vi "CSDB_SVEdit.main.vi"() -> ()   [LabVIEW 2014, in "CSDB_SVEdit.lvlib"]
doc: "Main VI of the Shared Variable Editor"
uses:
  CSDB_SVEdit.lvlib
panel:
  in  "dryRun":bool
  in  "showModifyProperty":bool
  in  "showSelected":bool
  in  "saveFile":bool
  in  "loadFile":bool
  in  "Undo":bool
  in  "doIt":bool
  in  "modifyValue":string
  in  "\"modifyValue\" preSelect":u16(ring)
  in  "usingAction":u16(ring)=3 items=["N/A", "append", "prefix", "replace"]
  in  "byValue":string
  in  "\"byValue\" preSelect":u16(ring)
  in  "modifyProperty":u16(ring)
  in  "\"selectValue\" preSelect":u16(ring)
  in  "selectValue":string
  in  "selectProperty":u16(ring)
  in  "sharedVariables":string[][](table)
  in  "exit":bool
  out "error out":errorcluster
  in  "error in (no error)":errorcluster
  in  "CSVPath":path
  # "if"
  # "Use \"selectProperty\" and \n\"selectName\" to select \nShared Variables (ROWS)"
  # "Use \"modifyProperty\" and \n\"modifyName\" to select values\nfor change (CELLS in a COLUMN)"
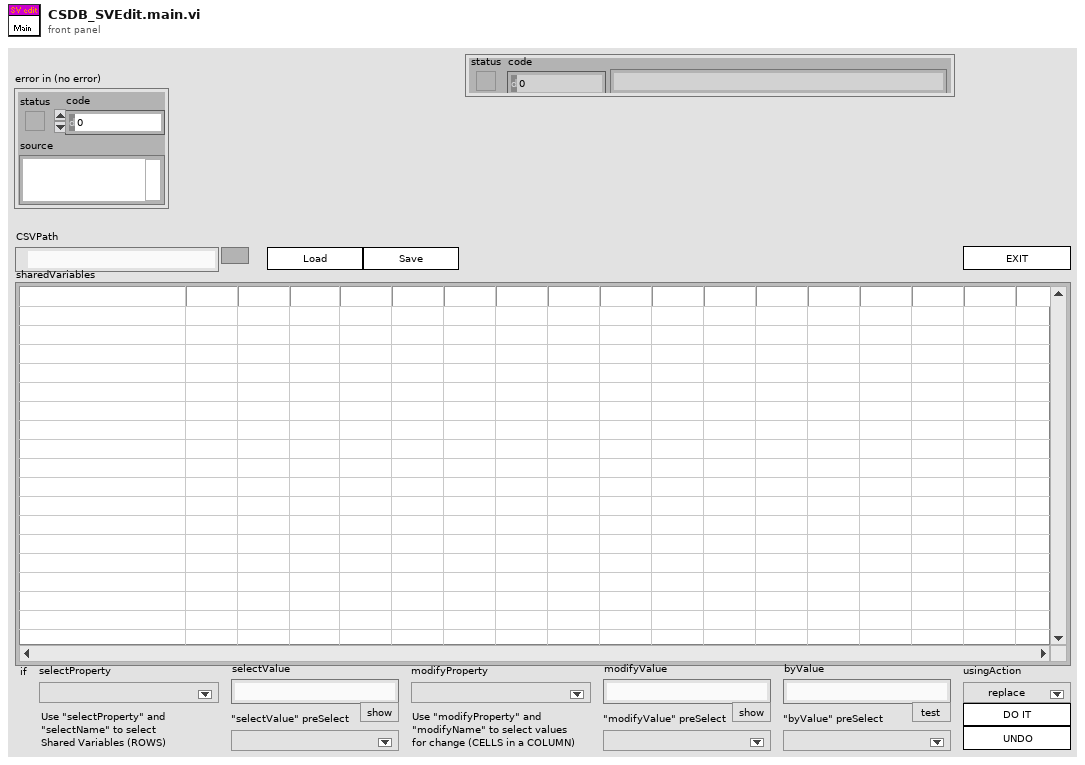
[diagram p1: front panel]
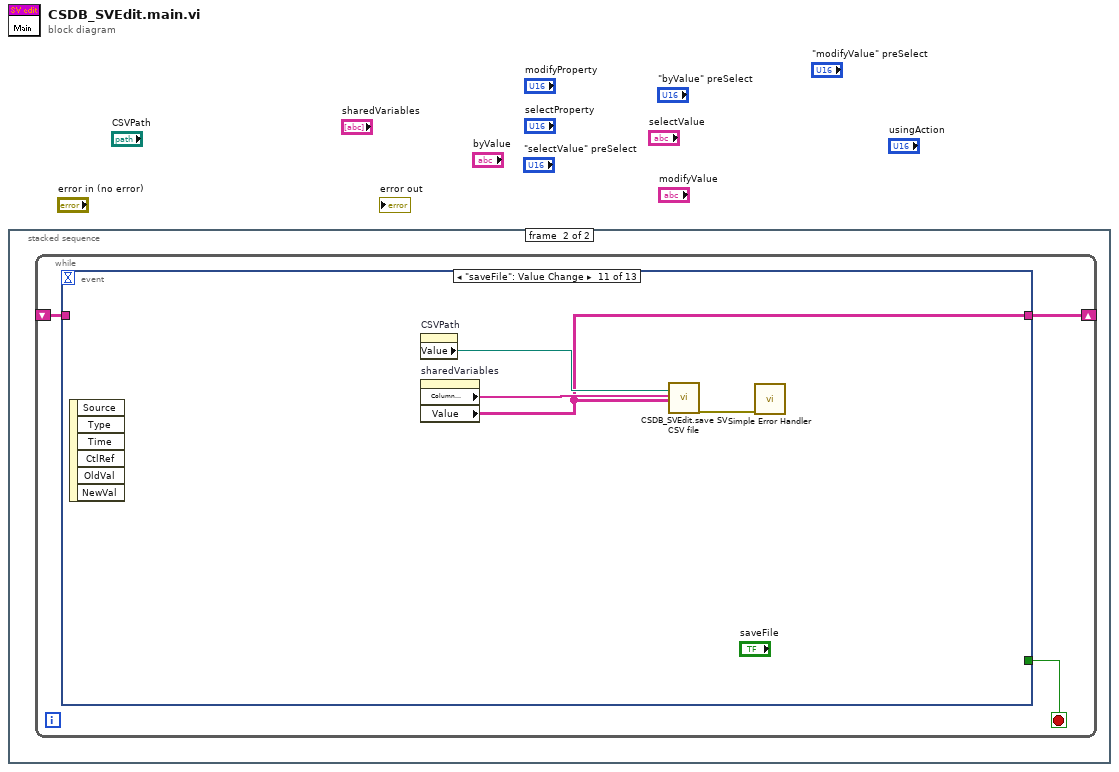
[diagram p0: block diagram]
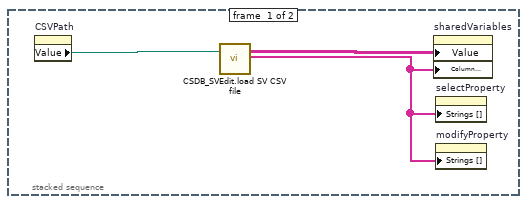
[diagram p2: hidden frame]
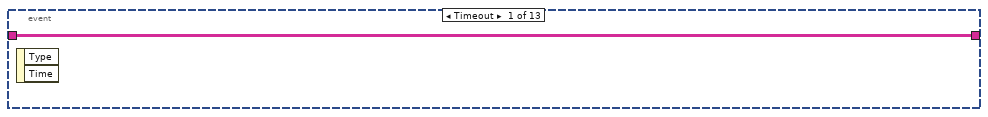
[diagram p3: hidden frame]
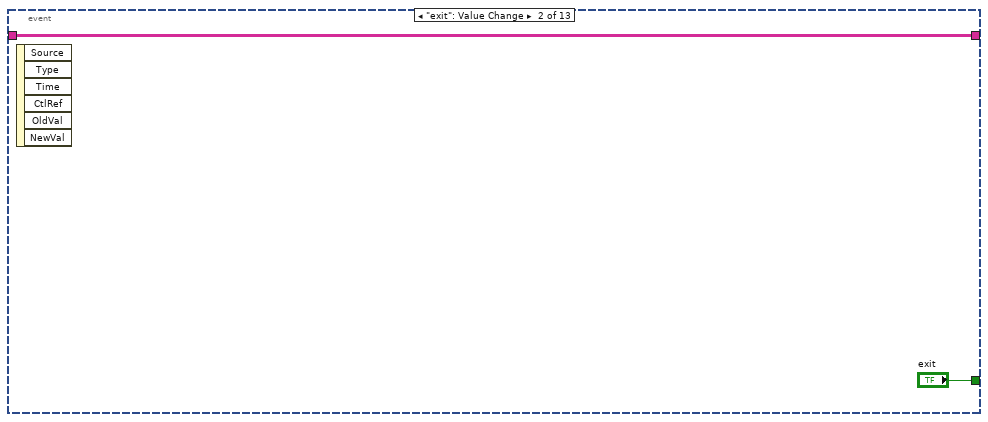
[diagram p4: hidden frame]
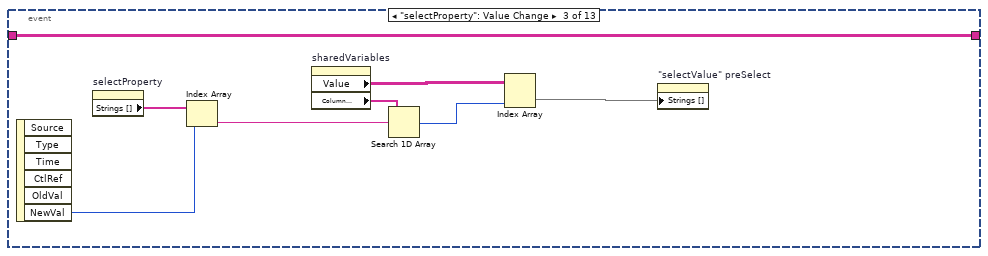
[diagram p5: hidden frame]
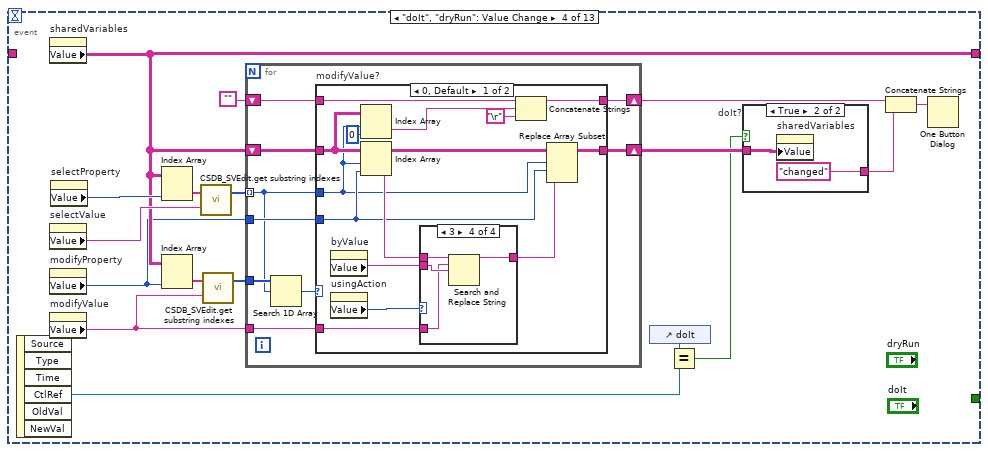
[diagram p6: hidden frame]
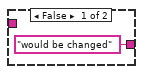
[diagram p7: hidden frame]
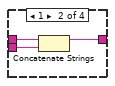
[diagram p9: hidden frame]
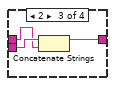
[diagram p10: hidden frame]
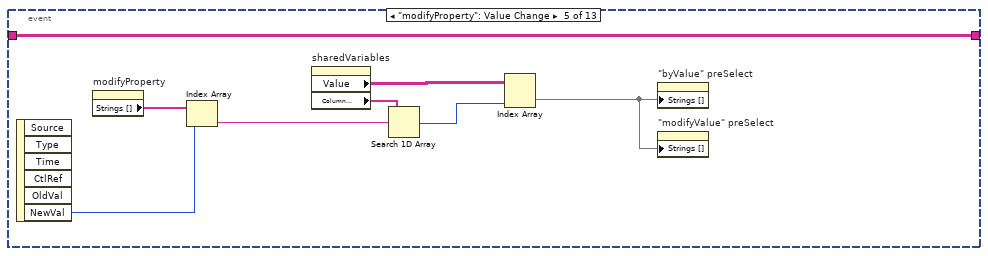
[diagram p12: hidden frame]
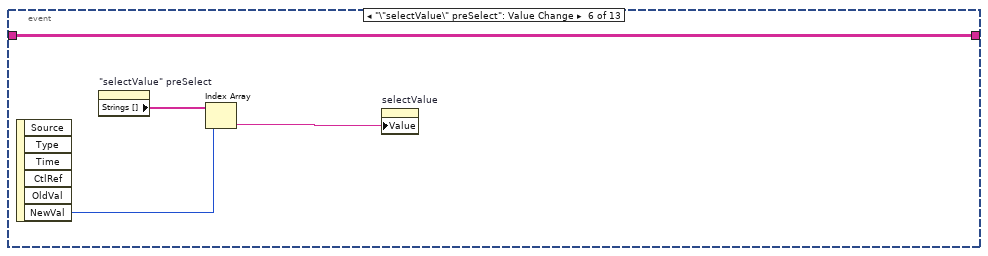
[diagram p13: hidden frame]
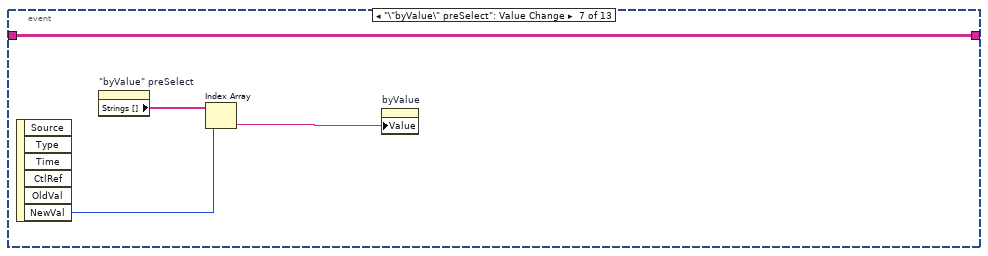
[diagram p14: hidden frame]
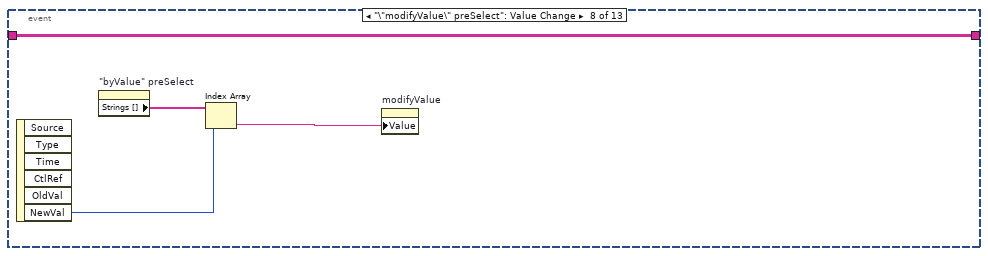
[diagram p15: hidden frame]
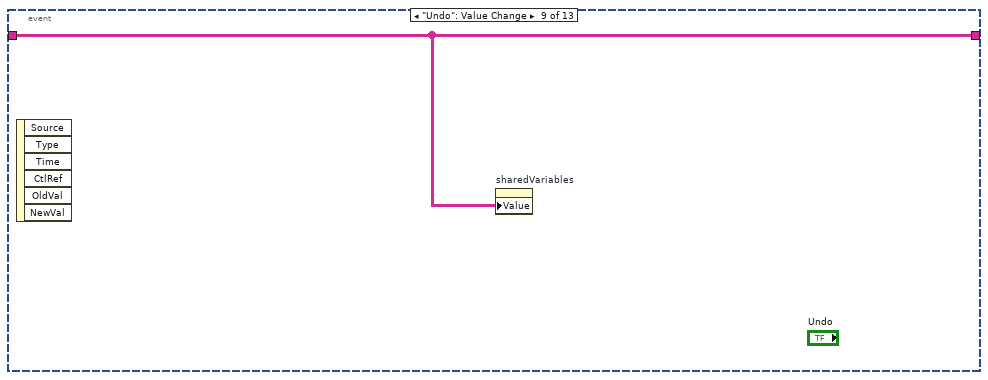
[diagram p16: hidden frame]
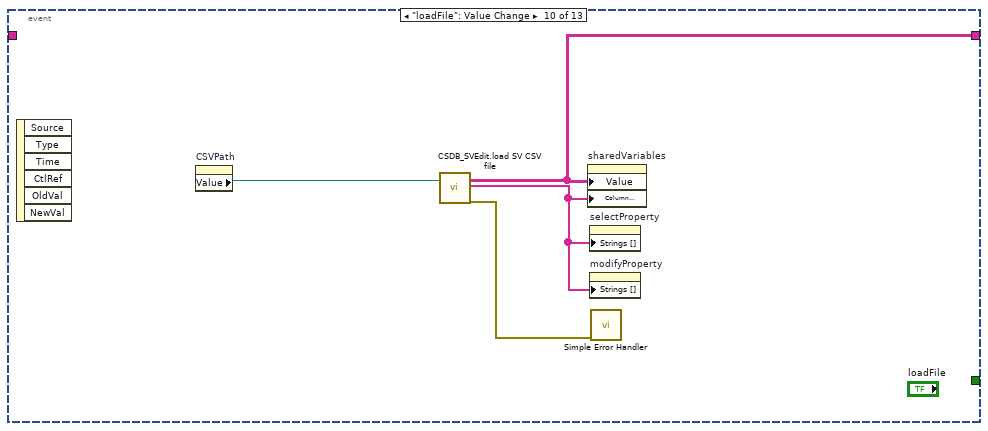
[diagram p17: hidden frame]
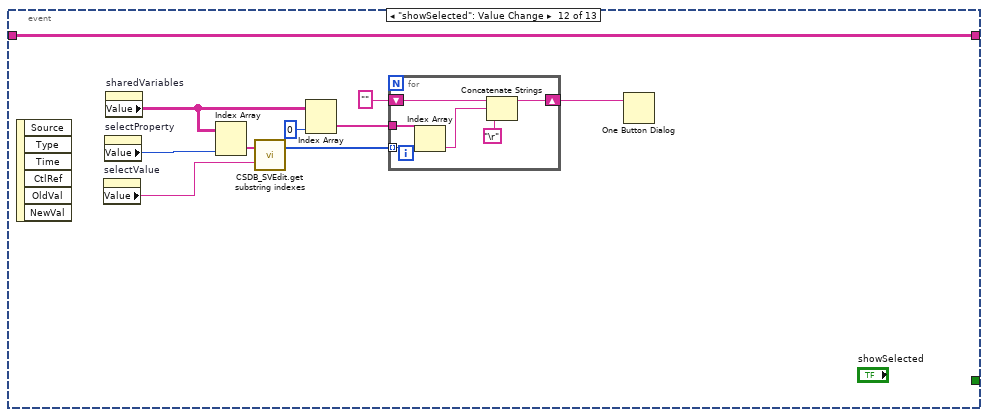
[diagram p18: hidden frame]
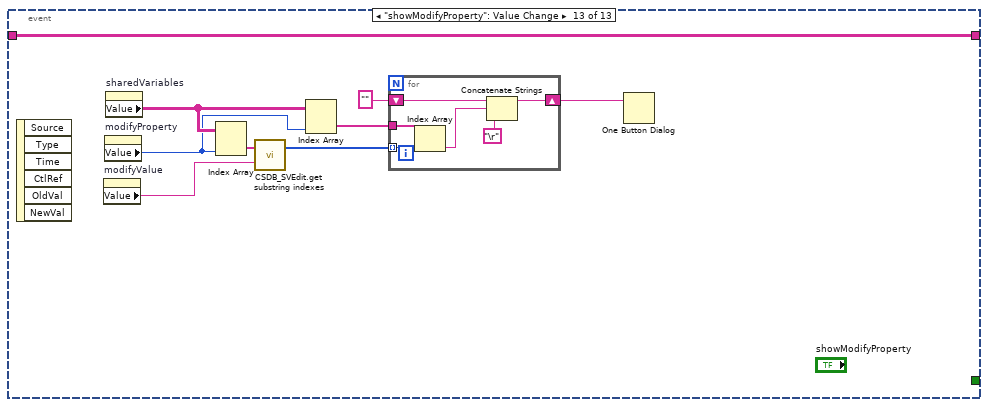
[diagram p19: hidden frame]
diagram:
  n1 = stacked-sequence {
    frame #0 {
      n2 = property on="CSVPath" class="Path"() -> ("Value"=w1:path)  [unwired: 2 in, 2 out]
      n3 = call "CSDB_SVEdit.load SV CSV file.vi"("CSVPath"=w1) -> ("SVValues"=w3:string[][], "SVHeader"=w2:string[])  [unwired: 16 in, 1 out]
      n4 = property on="sharedVariables" class="Tbl (strict)"("Value"=w3, "Column Headers[]"=w2) -> ()  [unwired: 2 in, 2 out]
      n5 = property on="selectProperty" class="Ring (strict)"("Strings []"=w2) -> ()  [unwired: 2 in, 2 out]
      n6 = property on="modifyProperty" class="Ring (strict)"("Strings []"=w2) -> ()  [unwired: 2 in, 2 out]
    }
    frame #1 {
      n7 = while {
        shift-right: [w5] -> _
        shift-left: _ -> [w4]
        stop <- w6 stop-if-true
        n8 = event shown="[10] \"saveFile\": Value Change" {
          selector: _ -> [_ _ _ _ _ _ _ _ _ _ _ _ _]
          dyn-events: _ -> [_ _ _ _ _ _ _ _ _ _ _ _ _]
          timeout: _ -> [_ _ _ _ _ _ _ _ _ _ _ _ _]
          tunnel: [_ "exit" _ _ _ _ _ _ _ _ _ _ _] -> w6
          tunnel: [w7 w8 w10 w28 w74 w82 w86 w90 w94 w96 w99 w112 w127] -> w5
          tunnel: w4 -> [w7 w8 w10 _ w74 w82 w86 w90 w94 _ _ w112 w127]
          event Timeout {
            n9 = event-data() -> ()  [unwired: 1 in, 2 out]
          }
          event "exit": Value Change {
            n10 = event-data() -> ()  [unwired: 1 in, 6 out]
          }
          event "selectProperty": Value Change {
            n11 = event-data() -> ("NewVal"=w16:u16)  [unwired: 1 in, 5 out]
            n12 = property on="selectProperty" class="Ring (strict)"() -> ("Strings []"=w17:string[])  [unwired: 2 in, 2 out]
            n13 = Index Array(array=w17, index=w16) -> (element=w15:string)
            n14 = property on="sharedVariables" class="Tbl (strict)"() -> ("Value"=w13:string[][], "Column Headers[]"=w14:string[])  [unwired: 2 in, 2 out]
            n15 = Search 1D Array(1D array=w14, element=w15) -> (index of element=w12:i32)  [unwired: 1 in]
            n16 = Index Array(array=w13, index (col)=w12) -> (element=w11:string[])  [unwired: 1 in]
            n17 = property on="\"selectValue\" preSelect" class="Ring (strict)"("Strings []"=w11) -> ()  [unwired: 2 in, 2 out]
          }
          event "doIt", "dryRun": Value Change {
            n18 = event-data() -> ("CtlRef"=w23:refnum<vi>)  [unwired: 1 in, 5 out]
            n19 = property on="sharedVariables" class="Tbl (strict)"() -> ("Value"=w28:string[][])  [unwired: 2 in, 2 out]
            n20 = property on="selectValue" class="Str"() -> ("Value"=w32:string)  [unwired: 2 in, 2 out]
            n21 = property on="modifyProperty" class="Ring (strict)"() -> ("Value"=w27:u16)  [unwired: 2 in, 2 out]
            n22 = property on="modifyValue" class="Str"() -> ("Value"=w26:string)  [unwired: 2 in, 2 out]
            n23 = property on="selectProperty" class="Ring (strict)"() -> ("Value"=w34:u16)  [unwired: 2 in, 2 out]
            n24 = Index Array(array=w28, index (col)=w34) -> (element=w33:string[])  [unwired: 1 in]
            n25 = Index Array(array=w28, index (col)=w27) -> (element=w30:string[])  [unwired: 1 in]
            n26 = call "CSDB_SVEdit.get substring indexes.vi"("stringArray"=w33, "subString"=w32) -> ("indexes"=w31:i32[])  [unwired: 17 in]
            n27 = call "CSDB_SVEdit.get substring indexes.vi"("stringArray"=w30, "subString"=w26) -> ("indexes"=w29:i32[])  [unwired: 17 in]
            n28 = for {
              tunnel: w31 -> [w42] mode=indexing
              tunnel: w29 -> [w43]
              tunnel: w27 -> [w44]
              tunnel: w26 -> [w41]
              shift-right: [w40] -> w25
              shift-left: w28 -> [w45]
              shift-right: [w38] -> w20
              shift-left: "" -> [w39]
              n29 = Search 1D Array(1D array=w43, element=w42) -> (index of element=w46:i32)  [unwired: 1 in]
              n30 = case "modifyValue?" shown="0, Default" w46 {
                tunnel: w45 -> [w53 w73]
                tunnel: w42 -> [w52 _]
                tunnel: w44 -> [w59 _]
                tunnel: w41 -> [w55 _]
                tunnel: [w54 w73] -> w40
                tunnel: w39 -> [w50 w72]
                tunnel: [w48 w72] -> w38
                frame 0, Default {
                  n31 = property on="byValue" class="Str"() -> ("Value"=w56:string)  [unwired: 2 in, 2 out]
                  n32 = property on="usingAction" class="Ring (strict)"() -> ("Value"=w58:u16)  [unwired: 2 in, 2 out]
                  n33 = Index Array(array=w53, index (row)=w52, index (col)=0 ("disabled index (col)")) -> (element=w49:string)
                  n34 = Index Array(array=w53, index (row)=w52, index (col)=w59) -> (element=w60:string)
                  n35 = case shown="3" w58 {
                    tunnel: w60 -> [w61 w64 w65 w71]
                    tunnel: [w61 w63 w67 w68] -> w57
                    tunnel: w56 -> [_ w62 w66 w70]
                    tunnel: w55 -> [_ _ _ w69]
                    frame 0, Default {
                    }
                    frame 1 {
                      n36 = Concatenate Strings(w64, w62) -> (w63:string)
                    }
                    frame 2 {
                      n37 = Concatenate Strings(w66, w65) -> (w67:string)
                    }
                    frame 3 {
                      n38 = Search and Replace String(input string=w71, search string=w69, replace string=w70) -> (result string=w68:string)  [unwired: 5 in, 3 out]
                    }
                  }
                  n39 = Concatenate Strings(w50, w49, "\r") -> (w48:string)
                  n40 = Replace Array Subset(array=w53, new element=w57, index (row)=w52, index (col)=w59) -> (w54:string[][])
                }
                frame -1 {
                }
              }
            }
            n41 = control-ref of="doIt"() -> (w24:refnum<vi>)
            n42 = Equal?(x=w24, y=w23) -> (x = y?=w22:bool)
            n43 = case "doIt?" shown="True" w22 {
              tunnel: w25 -> [_ w37]
              tunnel: ["would be changed" "changed"] -> w19
              frame False {
              }
              frame True {
                n44 = property on="sharedVariables" class="Tbl (strict)"("Value"=w37) -> ()  [unwired: 2 in, 2 out]
              }
            }
            n45 = Concatenate Strings(w20, w19) -> (w18:string)
            n46 = One Button Dialog(message=w18) -> ()  [unwired: 1 in, 1 out]
          }
          event "modifyProperty": Value Change {
            n47 = event-data() -> ("NewVal"=w80:u16)  [unwired: 1 in, 5 out]
            n48 = property on="modifyProperty" class="Ring (strict)"() -> ("Strings []"=w81:string[])  [unwired: 2 in, 2 out]
            n49 = Index Array(array=w81, index=w80) -> (element=w79:string)
            n50 = property on="sharedVariables" class="Tbl (strict)"() -> ("Value"=w77:string[][], "Column Headers[]"=w78:string[])  [unwired: 2 in, 2 out]
            n51 = Search 1D Array(1D array=w78, element=w79) -> (index of element=w76:i32)  [unwired: 1 in]
            n52 = Index Array(array=w77, index (col)=w76) -> (element=w75:string[])  [unwired: 1 in]
            n53 = property on="\"byValue\" preSelect" class="Ring (strict)"("Strings []"=w75) -> ()  [unwired: 2 in, 2 out]
            n54 = property on="\"modifyValue\" preSelect" class="Ring (strict)"("Strings []"=w75) -> ()  [unwired: 2 in, 2 out]
          }
          event "\"selectValue\" preSelect": Value Change {
            n55 = event-data() -> ("NewVal"=w84:u16)  [unwired: 1 in, 5 out]
            n56 = property on="\"selectValue\" preSelect" class="Ring (strict)"() -> ("Strings []"=w85:string[])  [unwired: 2 in, 2 out]
            n57 = Index Array(array=w85, index=w84) -> (element=w83:string)
            n58 = property on="selectValue" class="Str"("Value"=w83) -> ()  [unwired: 2 in, 2 out]
          }
          event "\"byValue\" preSelect": Value Change {
            n59 = event-data() -> ("NewVal"=w88:u16)  [unwired: 1 in, 5 out]
            n60 = property on="\"byValue\" preSelect" class="Ring (strict)"() -> ("Strings []"=w89:string[])  [unwired: 2 in, 2 out]
            n61 = Index Array(array=w89, index=w88) -> (element=w87:string)
            n62 = property on="byValue" class="Str"("Value"=w87) -> ()  [unwired: 2 in, 2 out]
          }
          event "\"modifyValue\" preSelect": Value Change {
            n63 = event-data() -> ("NewVal"=w92:u16)  [unwired: 1 in, 5 out]
            n64 = property on="\"byValue\" preSelect" class="Ring (strict)"() -> ("Strings []"=w93:string[])  [unwired: 2 in, 2 out]
            n65 = Index Array(array=w93, index=w92) -> (element=w91:string)
            n66 = property on="modifyValue" class="Str"("Value"=w91) -> ()  [unwired: 2 in, 2 out]
          }
          event "Undo": Value Change {
            n67 = event-data() -> ()  [unwired: 1 in, 6 out]
            n68 = property on="sharedVariables" class="Tbl (strict)"("Value"=w94) -> ()  [unwired: 2 in, 2 out]
          }
          event "loadFile": Value Change {
            n69 = event-data() -> ()  [unwired: 1 in, 6 out]
            n70 = property on="CSVPath" class="Path"() -> ("Value"=w98:path)  [unwired: 2 in, 2 out]
            n71 = call "CSDB_SVEdit.load SV CSV file.vi"("CSVPath"=w98) -> ("SVValues"=w96:string[][], "SVHeader"=w97:string[], "error out"=w95:errorcluster)  [unwired: 16 in]
            n72 = property on="sharedVariables" class="Tbl (strict)"("Value"=w96, "Column Headers[]"=w97) -> ()  [unwired: 2 in, 2 out]
            n73 = property on="selectProperty" class="Ring (strict)"("Strings []"=w97) -> ()  [unwired: 2 in, 2 out]
            n74 = property on="modifyProperty" class="Ring (strict)"("Strings []"=w97) -> ()  [unwired: 2 in, 2 out]
            n75 = call <vilib>:"Simple Error Handler.vi"("error in (no error)"=w95) -> ()  [unwired: 4 in, 5 out]
          }
          event "saveFile": Value Change {
            n76 = event-data() -> ()  [unwired: 1 in, 6 out]
            n77 = property on="CSVPath" class="Path"() -> ("Value"=w101:path)  [unwired: 2 in, 2 out]
            n78 = property on="sharedVariables" class="Tbl (strict)"() -> ("Column Headers[]"=w102:string[], "Value"=w99:string[][])  [unwired: 2 in, 2 out]
            n79 = call "CSDB_SVEdit.save SV CSV file.vi"("CSVPath"=w101, "SVHeader"=w102, "SVValues"=w99) -> ("error out"=w100:errorcluster)  [unwired: 16 in]
            n80 = call <vilib>:"Simple Error Handler.vi"("error in (no error)"=w100) -> ()  [unwired: 4 in, 5 out]
          }
          event "showSelected": Value Change {
            n81 = event-data() -> ()  [unwired: 1 in, 6 out]
            n82 = property on="selectValue" class="Str"() -> ("Value"=w109:string)  [unwired: 2 in, 2 out]
            n83 = property on="selectProperty" class="Ring (strict)"() -> ("Value"=w111:u16)  [unwired: 2 in, 2 out]
            n84 = property on="sharedVariables" class="Tbl (strict)"() -> ("Value"=w108:string[][])  [unwired: 2 in, 2 out]
            n85 = Index Array(array=w108, index (col)=w111) -> (element=w110:string[])  [unwired: 1 in]
            n86 = call "CSDB_SVEdit.get substring indexes.vi"("stringArray"=w110, "subString"=w109) -> ("indexes"=w105:i32[])  [unwired: 17 in]
            n87 = Index Array(array=w108, index (col)=0 ("disabled index (col)")) -> (element=w106:string[])  [unwired: 1 in]
            n88 = for {
              tunnel: w106 -> [w116]
              tunnel: w105 -> [w117] mode=indexing
              shift-right: [w113] -> w103
              shift-left: "" -> [w118]
              n89 = Index Array(array=w116, index=w117) -> (element=w115:string)
              n90 = Concatenate Strings(w118, w115, "\r") -> (w113:string)
            }
            n91 = One Button Dialog(message=w103) -> ()  [unwired: 1 in, 1 out]
          }
          event "showModifyProperty": Value Change {
            n92 = event-data() -> ()  [unwired: 1 in, 6 out]
            n93 = property on="modifyValue" class="Str"() -> ("Value"=w125:string)  [unwired: 2 in, 2 out]
            n94 = property on="modifyProperty" class="Ring (strict)"() -> ("Value"=w119:u16)  [unwired: 2 in, 2 out]
            n95 = property on="sharedVariables" class="Tbl (strict)"() -> ("Value"=w124:string[][])  [unwired: 2 in, 2 out]
            n96 = Index Array(array=w124, index (col)=w119) -> (element=w126:string[])  [unwired: 1 in]
            n97 = call "CSDB_SVEdit.get substring indexes.vi"("stringArray"=w126, "subString"=w125) -> ("indexes"=w122:i32[])  [unwired: 17 in]
            n98 = Index Array(array=w124, index (col)=w119) -> (element=w123:string[])  [unwired: 1 in]
            n99 = for {
              tunnel: w123 -> [w131]
              tunnel: w122 -> [w132] mode=indexing
              shift-right: [w128] -> w120
              shift-left: "" -> [w133]
              n100 = Index Array(array=w131, index=w132) -> (element=w130:string)
              n101 = Concatenate Strings(w133, w130, "\r") -> (w128:string)
            }
            n102 = One Button Dialog(message=w120) -> ()  [unwired: 1 in, 1 out]
          }
        }
      }
    }
  }
